vi "audio-stim-play.vi"(11 "Stimulus List":dbl[][](array[numeric])) -> (3 "Playing":bool caption="Playing stimulus")   [LabVIEW 2009]
uses:
  <vilib>/DAQmx/create/channels.llb/DAQmx Create Channel (DO-Digital Output).vi
  <vilib>/DAQmx/write.llb/DAQmx Write (Digital U16 1Chan 1Samp).vi
  <vilib>/DAQmx/create/channels.llb/DAQmx Create Channel (AO-Voltage-Basic).vi
  <vilib>/DAQmx/configure/timing.llb/DAQmx Timing (Use Waveform).vi
  <vilib>/DAQmx/write.llb/DAQmx Write (Analog Wfm 1Chan NSamp).vi
panel:
  out "Log File Path":path
  in  "Play Interval Jitter (s)":dbl
  in  "Play Interval (s)":dbl
  out "error out":errorcluster
  in  "DO Ports":tag caption="DO Ports\n(\"browse\" and select two 8 bit ports)"
  in  "Sound AO Channel":tag
  out "Curr Param":dbl[](array[numeric]) caption="Current (or Cued) Trial Parameters"
  in  "Sampling Rate":dbl
  in  "stop":bool
  in  "Play":bool
  out "Current (or Cued) Waveform":waveform(dbl)(graph)
  out "Waiting":bool
  in  "Current (or Cued) Trial":i32(slide) min=0 max=20
  # "Stim#, Stim Type, Duration, Amplitude, Param 1, Param 2, Param 3, Param 4"
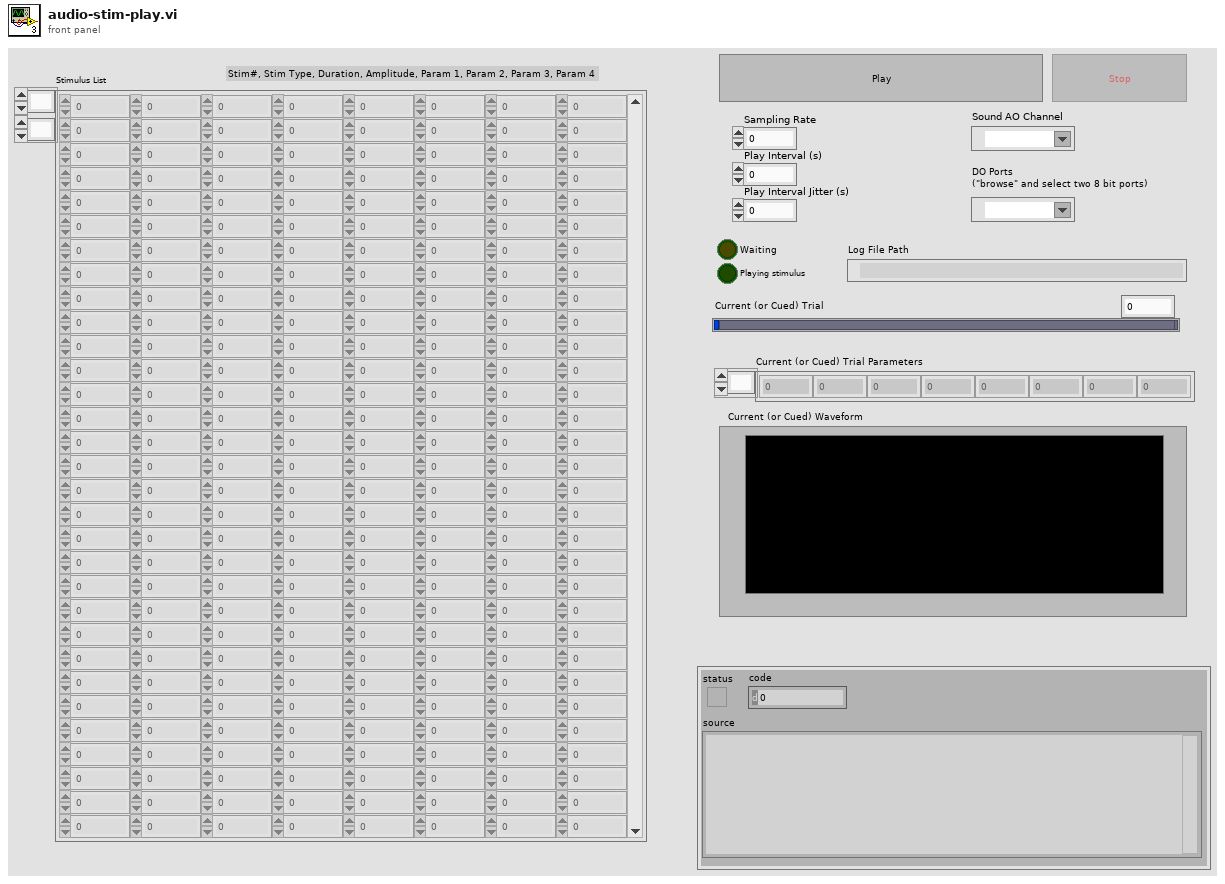
[diagram p1: front panel]
types:
  T1 = cluster{"Sampling Rate":dbl, "Value 3":dbl, dbl, "Value 2":dbl}
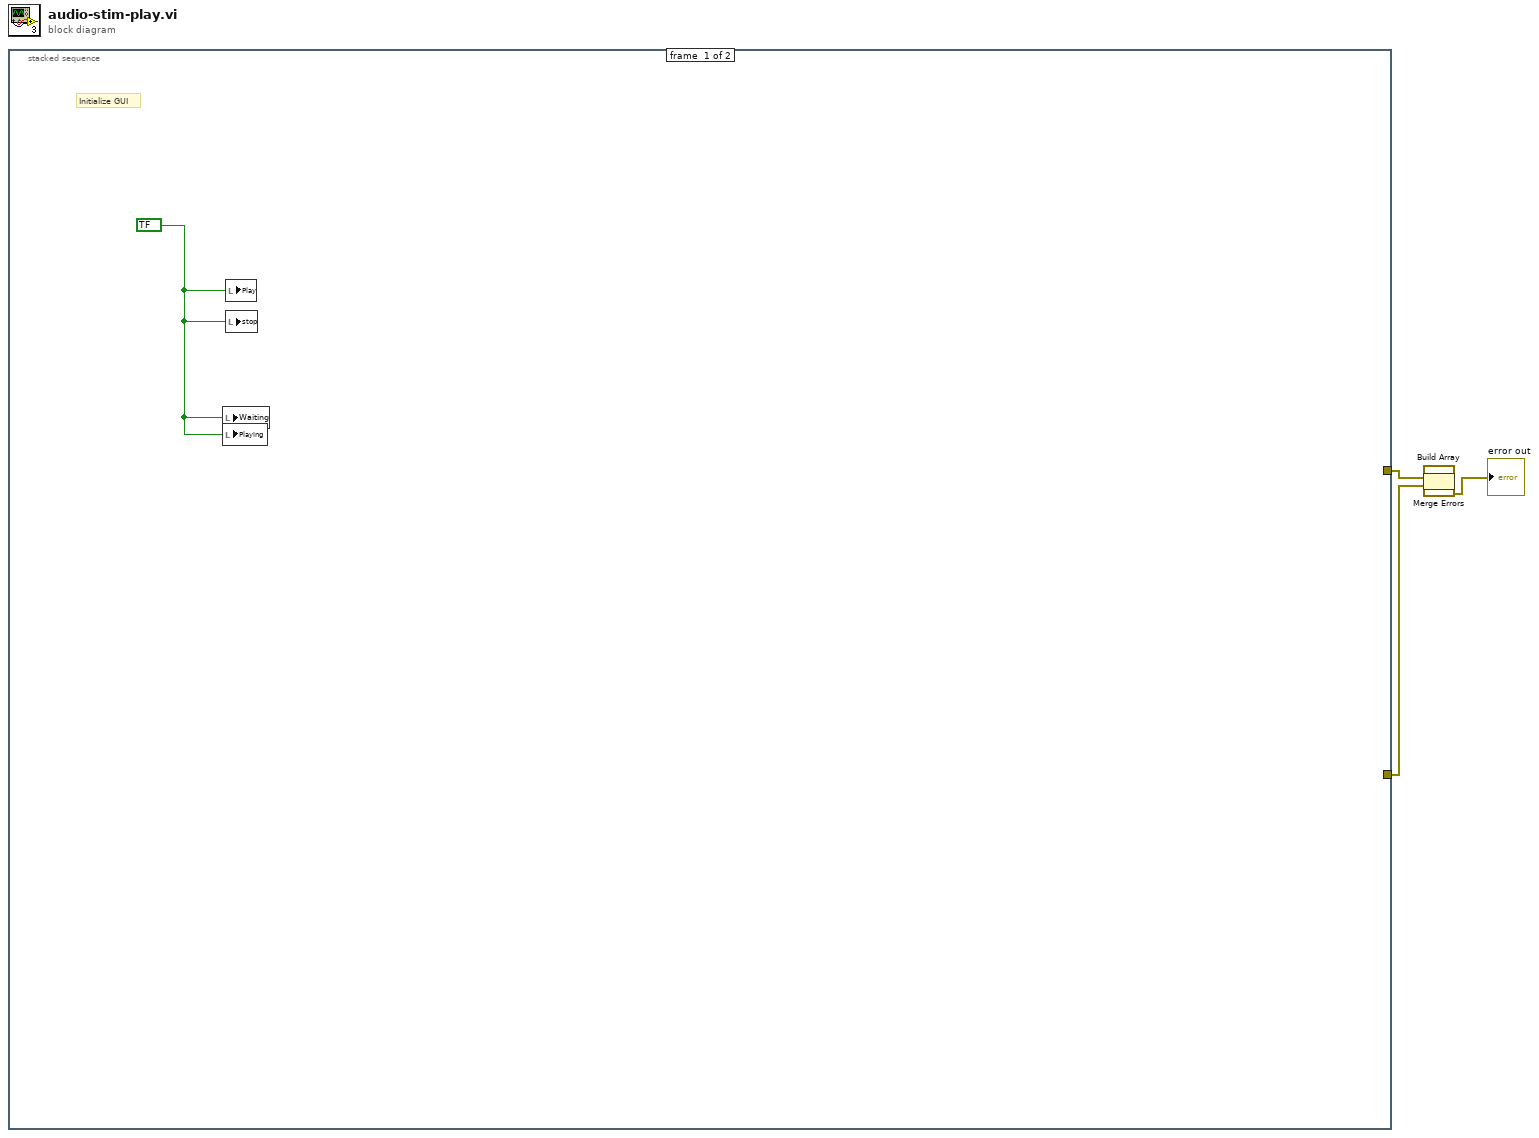
[diagram p0: block diagram]
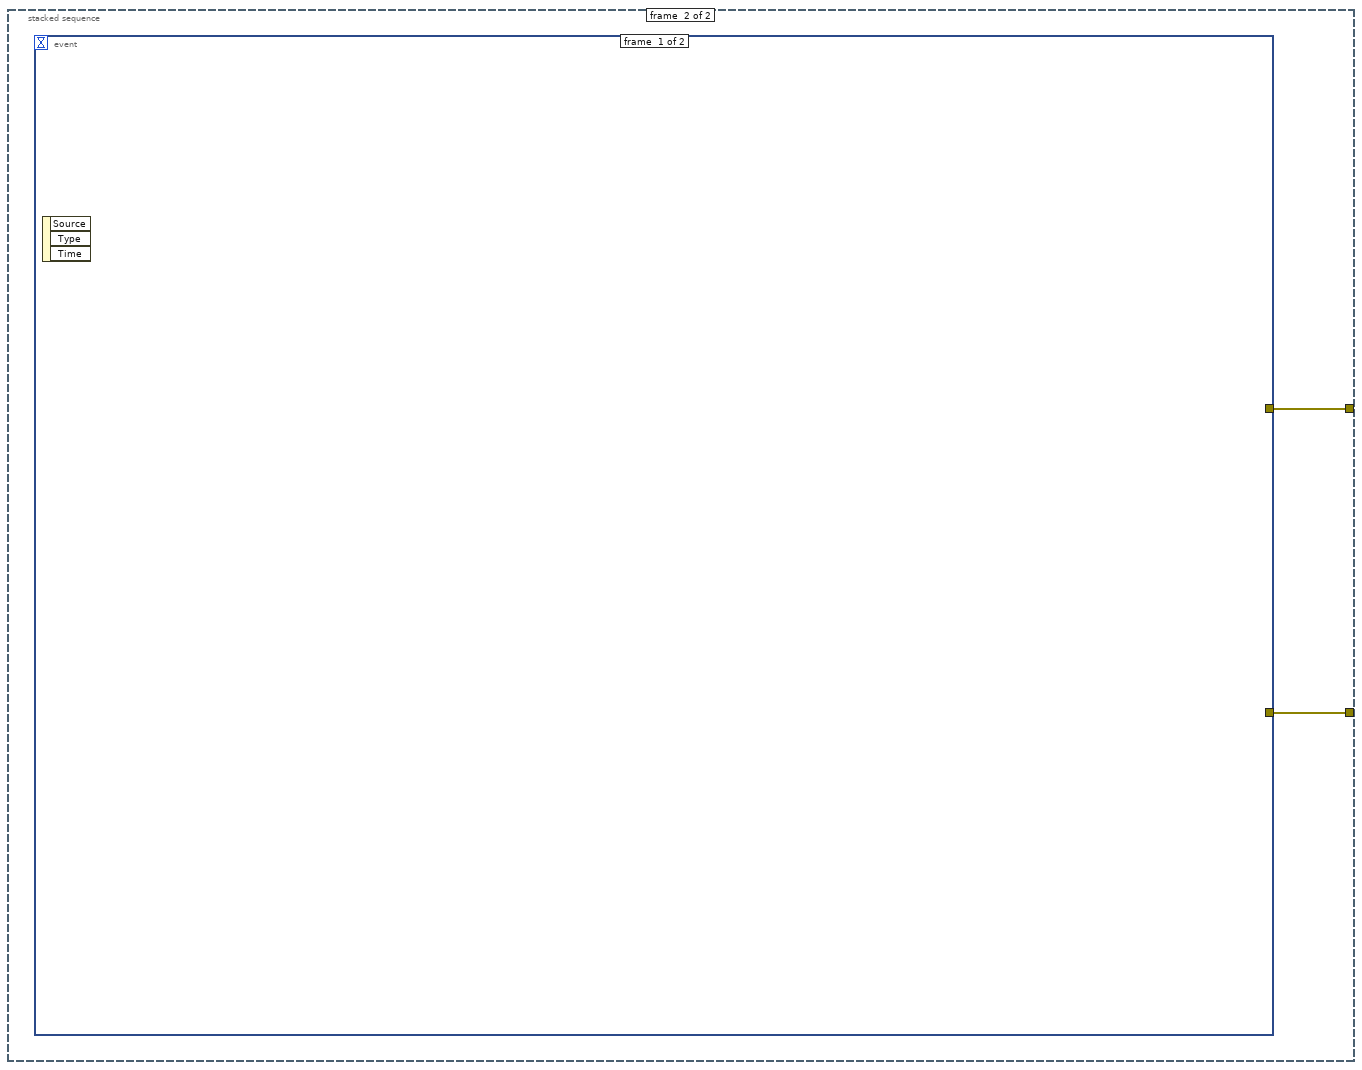
[diagram p2: hidden frame]
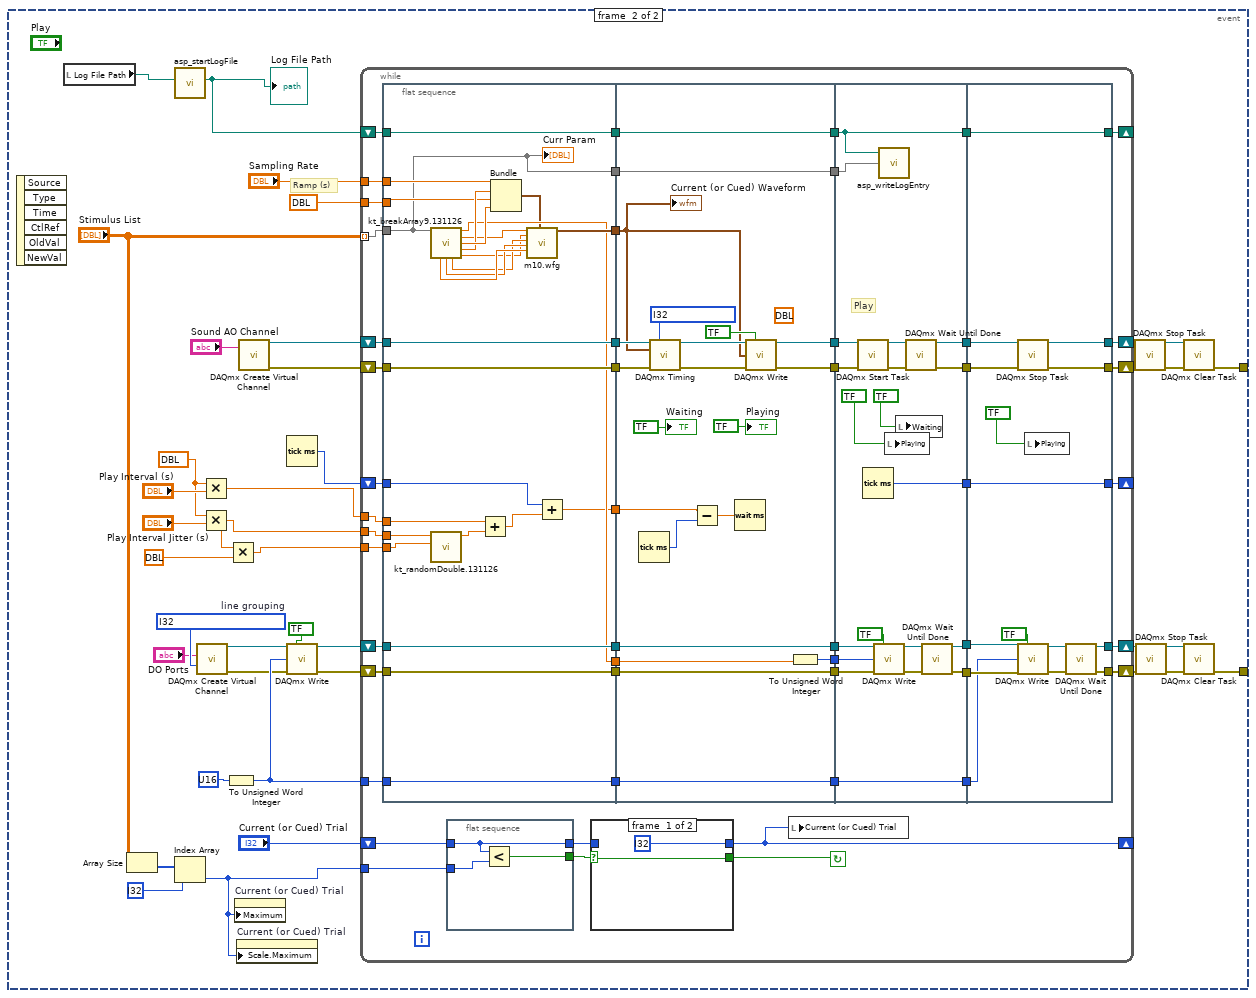
[diagram p3: hidden frame]
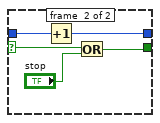
[diagram p4: hidden frame]
diagram:
  n1 = stacked-sequence {
    tunnel: [_ w7] -> w4
    tunnel: [_ w6] -> w3
    frame #0 {
      w5 = bool ? ("Play")
      # "Initialize GUI"
      n2 = local write "Waiting"(w5) -> ()
      n3 = local write "Playing"(w5) -> ()
      n4 = local write "Play"(w5) -> ()
      n5 = local write "stop"(w5) -> ()
    }
    frame #1 {
      n6 = event shown="[1] \"Play\": Value Change" {
        selector: _ -> [_ _]
        dyn-events: _ -> [_ _]
        timeout: _ -> [_ _]
        tunnel: [_ w22] -> w7
        tunnel: [_ w21] -> w6
        event #0 {
          n7 = event-data() -> ()  [unwired: 1 in, 3 out]
        }
        event #1 {
          w14 = dbl ? ("y")
          w43 = i32 ? items=["one channel for each line", "one channel for all lines"]  # line grouping
          # "Ramp (s)"
          n8 = event-data() -> ()  [unwired: 1 in, 6 out]
          n9 = local read "Log File Path"() -> (w9:path)
          n10 = Array Size(array="Stimulus List") -> (size(s)=w41:i32[])
          n11 = call "asp_startLogFile.vi"("Path In"=w9) -> ("Path"=w8:path)  [unwired: 5 in, 1 out]
          "Log File Path" <- w8
          n12 = Index Array(array=w41, index=i32 ?) -> (element=w25:i32)
          n13 = call-poly <vilib>:"DAQmx Create Virtual Channel.vi"("lines"="DO Ports", "line grouping"=w43) -> ("task out"=w19:refnum<k21>, "error out"=w18:errorcluster)  [unwired: 12 in]
          n14 = Multiply(x=w14, y="Play Interval (s)") -> (x*y=w13:dbl)
          n15 = Multiply(x=w14, y="Play Interval Jitter (s)") -> (x*y=w11:dbl)
          n16 = To Unsigned Word Integer(number=u16 ? ("data")) -> (unsigned 16bit integer=w26:u16)
          n17 = Multiply(x=w11, y=dbl ?) -> (x*y=w12:dbl)
          n18 = property on="Current (or Cued) Trial" class="Slide (strict)"("Maximum"=w25) -> ()  [unwired: 2 in, 2 out]
          n19 = property on="Current (or Cued) Trial" class="Slide (strict)"("Scale.Maximum"=w25) -> ()  [unwired: 2 in, 2 out]
          n20 = call-poly <vilib>:"DAQmx Create Virtual Channel.vi"("physical channels"="Sound AO Channel") -> ("task out"=w24:refnum<k21>, "error out"=w23:errorcluster)  [unwired: 13 in]
          n21 = Tick Count (ms)() -> (millisecond timer value=w10:u32)
          n22 = call-poly <vilib>:"DAQmx Write.vi"("task/channels in"=w19, "auto start"=bool ?, "data"=w26, "error in"=w18) -> ("task out"=w30:refnum<k21>, "error out"=w29:errorcluster)  [unwired: 9 in, 1 out]
          n23 = while {
            tunnel: "Stimulus List" -> [w64] mode=indexing
            tunnel: "Sampling Rate" -> [w63]
            tunnel: dbl ? -> [w62]
            shift-right: [w94] -> w35
            shift-left: w24 -> [w92]
            shift-right: [w93] -> w34
            shift-left: w23 -> [w91]
            shift-right: [w81] -> w39
            shift-left: w30 -> [w90]
            shift-right: [w80] -> w38
            shift-left: w29 -> [w72]
            shift-right: [w75] -> _
            shift-left: "Current (or Cued) Trial" -> [w84]
            tunnel: w25 -> [w83]
            tunnel: w26 -> [w78]
            shift-right: [w59] -> _
            shift-left: w10 -> [w58]
            tunnel: w13 -> [w54]
            tunnel: w12 -> [w55]
            tunnel: w11 -> [w56]
            shift-right: [w47] -> _
            shift-left: w8 -> [w53]
            stop <- w73 continue-if-true
            n24 = flat-sequence {
              tunnel: w72 -> [w128]
              tunnel: w78 -> [w129]
              tunnel: w90 -> [w130]
              tunnel: w91 -> [w131]
              tunnel: w92 -> [w132]
              tunnel: [w132] -> w70
              tunnel: [w131] -> w69
              tunnel: [w130] -> w68
              tunnel: [w129] -> w67
              tunnel: [w128] -> w66
              tunnel: [w120] -> w65
              tunnel: w64 -> [w107]
              tunnel: w63 -> [w119]
              tunnel: w62 -> [w118]
              tunnel: [w117] -> w61
              tunnel: w58 -> [w115]
              tunnel: [w114] -> w57
              tunnel: w56 -> [w113]
              tunnel: w55 -> [w112]
              tunnel: w54 -> [w109]
              tunnel: w53 -> [w108]
              tunnel: [w108] -> w52
              tunnel: [w107] -> w51
              tunnel: [w143] -> w96
              tunnel: [w142] -> w95
              tunnel: [w152] -> w89
              tunnel: [w151] -> w82
              tunnel: [w150] -> w79
              tunnel: [w140] -> w71
              tunnel: w70 -> [w149]
              tunnel: w69 -> [w148]
              tunnel: w68 -> [w152]
              tunnel: w67 -> [w150]
              tunnel: w66 -> [w140]
              tunnel: w65 -> [w139]
              tunnel: w61 -> [w138]
              tunnel: w57 -> [w135]
              tunnel: w52 -> [w133]
              tunnel: w51 -> [w134]
              tunnel: [w134] -> w50
              tunnel: [w133] -> w49
              tunnel: w96 -> [w163]
              tunnel: w95 -> [w162]
              tunnel: w89 -> [w171]
              tunnel: [w165] -> w88
              tunnel: [w164] -> w87
              tunnel: [w168] -> w86
              tunnel: [w167] -> w85
              tunnel: w82 -> [w172]
              tunnel: w79 -> [w166]
              tunnel: [w166] -> w77
              tunnel: w71 -> [w157]
              tunnel: [w156] -> w60
              tunnel: w50 -> [w155]
              tunnel: w49 -> [w154]
              tunnel: [w154] -> w48
              tunnel: [w176] -> w93
              tunnel: [w177] -> w94
              tunnel: w88 -> [w179]
              tunnel: w87 -> [w178]
              tunnel: w86 -> [w187]
              tunnel: w85 -> [w186]
              tunnel: [w182] -> w81
              tunnel: [w181] -> w80
              tunnel: w77 -> [w180]
              tunnel: w60 -> [w175]
              tunnel: [w175] -> w59
              tunnel: w48 -> [w174]
              tunnel: [w174] -> w47
              frame #0 {
                n25 = call "kt_breakArray9.131126.vi"("Current (or Cued Trial Parameters)"=w107) -> ("Value 0"=w117:dbl, "Value 1"=w121:dbl, "Value 2"=w123:dbl, "Value 3"=w122:dbl, "Value 7"=w127:dbl, "Value 6"=w126:dbl, "Value 5"=w125:dbl, "Value 4"=w124:dbl)  [unwired: 6 in, 1 out]
                n26 = call "kt_randomDouble.131126.vi"("Min"=w112, "Max"=w113) -> ("Random"=w110:dbl)  [unwired: 9 in]
                n27 = Add(x=w109, y=w110) -> (x+y=w111:dbl)
                n28 = Bundle("Sampling Rate"=w119, "Value 3"=w122, w118, "Value 2"=w123) -> (w116:T1)  [unwired: 1 in]
                n29 = call "m10.wfg.vi"("Stimulus Type"=w121, "Param 0"=w124, "Param 1"=w125, "Param 2"=w126, "Param 3"=w127, "Waveform Properties"=w116) -> ("Waveform Out"=w120:waveform(dbl))  [unwired: 12 in, 1 out]
                n30 = Add(x=w115, y=w111) -> (x+y=w114:dbl)
                "Curr Param" <- w107
              }
              frame #1 {
                (unwired) dbl ? ("timeout")
                w147 = i32 ? items=["Finite Samples", "Continuous Samples", "Hardware Timed Single Point"] ("sample mode")
                n31 = Tick Count (ms)() -> (millisecond timer value=w136:u32)
                n32 = call-poly <vilib>:"DAQmx Timing.vi"("task/channels in"=w149, "sample mode"=w147, "waveform"=w139, "error in"=w148) -> ("task out"=w146:refnum<k21>, "error out"=w145:errorcluster)  [unwired: 10 in]
                n33 = Subtract(x=w135, y=w136) -> (x-y=w137:dbl)
                n34 = Wait (ms)(milliseconds to wait=w137) -> ()  [unwired: 1 out]
                n35 = call-poly <vilib>:"DAQmx Write.vi"("task/channels in"=w146, "auto start"=bool ?, "data"=w139, "error in"=w145) -> ("task out"=w143:refnum<k21>, "error out"=w142:errorcluster)  [unwired: 9 in, 1 out]
                n36 = To Unsigned Word Integer(number=w138) -> (unsigned 16bit integer=w151:u16)
                "Waiting" <- bool ? ("Playing Stimulus")
                "Playing" <- bool ? ("Playing Stimulus")
                "Current (or Cued) Waveform" <- w139
              }
              frame #2 {
                # "Play"
                n37 = call <vilib>:"DAQmx Start Task.vi"("task/channels in"=w163, "error in"=w162) -> ("task out"=w161:refnum<k21>, "error out"=w160:errorcluster)  [unwired: 12 in]
                n38 = Tick Count (ms)() -> (millisecond timer value=w156:u32)
                n39 = call-poly <vilib>:"DAQmx Write.vi"("task/channels in"=w171, "auto start"=bool ?, "data"=w172, "error in"=w157) -> ("task out"=w170:refnum<k21>, "error out"=w169:errorcluster)  [unwired: 9 in, 1 out]
                n40 = call "asp_writeLogEntry.vi"("Path In"=w154, "Curr Param"=w155) -> ()  [unwired: 4 in, 1 out]
                n41 = local write "Playing"(bool ? ("Playing Stimulus")) -> ()
                n42 = local write "Waiting"(bool ? ("Playing Stimulus")) -> ()
                n43 = call <vilib>:"DAQmx Wait Until Done.vi"("task/channels in"=w161, "error in"=w160) -> ("task out"=w165:refnum<k21>, "error out"=w164:errorcluster)  [unwired: 12 in]
                n44 = call <vilib>:"DAQmx Wait Until Done.vi"("task/channels in"=w170, "error in"=w169) -> ("task out"=w168:refnum<k21>, "error out"=w167:errorcluster)  [unwired: 12 in]
              }
              frame #3 {
                n45 = call <vilib>:"DAQmx Stop Task.vi"("task/channels in"=w179, "error in"=w178) -> ("task out"=w177:refnum<k21>, "error out"=w176:errorcluster)  [unwired: 12 in]
                n46 = call-poly <vilib>:"DAQmx Write.vi"("task/channels in"=w187, "auto start"=bool ?, "data"=w180, "error in"=w186) -> ("task out"=w184:refnum<k21>, "error out"=w183:errorcluster)  [unwired: 9 in, 1 out]
                n47 = local write "Playing"(bool ? ("Playing Stimulus")) -> ()
                n48 = call <vilib>:"DAQmx Wait Until Done.vi"("task/channels in"=w184, "error in"=w183) -> ("task out"=w182:refnum<k21>, "error out"=w181:errorcluster)  [unwired: 12 in]
              }
            }
            n49 = flat-sequence {
              tunnel: w84 -> [w104]
              tunnel: w83 -> [w106]
              tunnel: [w105] -> w74
              tunnel: [w104] -> w76
              frame #0 {
                n50 = Less?(x=w104, y=w106) -> (x < y?=w105:bool)
              }
            }
            n51 = case shown="True" w74 {
              selector: w74 -> [w97 w100]
              tunnel: w76 -> [_ w103]
              tunnel: [i32 ? w102] -> w75
              tunnel: [w97 w101] -> w73
              frame #0 {
              }
              frame #1 {
                n52 = Increment(x=w103) -> (x+1=w102:i32)
                n53 = Or(x=w100, y="stop") -> (x .or. y?=w101:bool)
              }
            }
            n54 = local write "Current (or Cued) Trial"(w75) -> ()
          }
          n55 = call <vilib>:"DAQmx Stop Task.vi"("task/channels in"=w35, "error in"=w34) -> ("task out"=w33:refnum<k21>, "error out"=w32:errorcluster)  [unwired: 12 in]
          n56 = call <vilib>:"DAQmx Stop Task.vi"("task/channels in"=w39, "error in"=w38) -> ("task out"=w37:refnum<k21>, "error out"=w36:errorcluster)  [unwired: 12 in]
          n57 = call <vilib>:"DAQmx Clear Task.vi"("task in"=w33, "error in"=w32) -> ("error out"=w22:errorcluster)  [unwired: 13 in]
          n58 = call <vilib>:"DAQmx Clear Task.vi"("task in"=w37, "error in"=w36) -> ("error out"=w21:errorcluster)  [unwired: 13 in]
        }
      }
    }
  }
  n59 = Build Array(w4, w3) -> (w1:errorcluster[])
  n60 = call <vilib>:"Merge Errors.vi"("error array in"=w1) -> ("error out"=→"error out":errorcluster)  [unwired: 6 in]
